vi "中英文全局.vi"() -> ()   [LabVIEW 2013]
panel:
  in  "中英文选择":enum32{"中文", "English"}(radio)
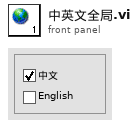
[diagram p1: front panel]
diagram:
